vi "SRsesnsitivityConversion5110.vi"(9 "Sen":dbl format="%#_13g", 11 "Input":dbl=0.00012) -> (3 "Output":dbl=0.00012)   [LabVIEW 2013]
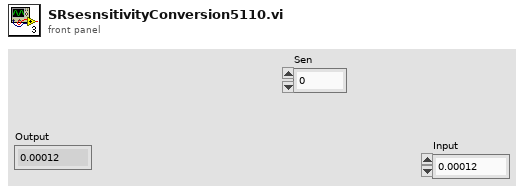
[diagram p1: front panel]
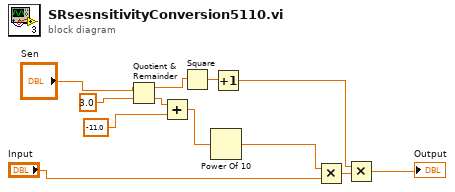
[diagram p0: block diagram]
diagram:
  n1 = Quotient & Remainder(x="Sen", y=3.0) -> (x-y*floor(x/y)=w5:dbl, floor(x/y)=w10:dbl)
  n2 = Add(x=w10, y=-11.0) -> (x+y=w8:dbl)
  n3 = Square(x=w5) -> (x^2=w4:dbl)
  n4 = Power Of 10(x=w8) -> (10^x=w7:dbl)
  n5 = Increment(x=w4) -> (x+1=w2:dbl)
  n6 = Multiply(x=w7, y="Input") -> (x*y=w3:dbl)
  n7 = Multiply(x=w2, y=w3) -> (x*y=→"Output":dbl)
